vi "Select PPMS Class.vi"(8 "error in (no error)":errorcluster, 11 "Select PPMS":T1) -> (0 "error out":errorcluster, 3 "instrument.PPMS out":refnum<class "instrument.PPMS.lvclass">)   [LabVIEW 2019, in "instrument.PPMS.lvclass"]
uses:
  instrument.PPMS.lvclass
  Typedefs/Select PPMS--Enum.ctl
  instrument.PPMS1/instrument.PPMS1.lvclass
  C:/Users/patrick/Documents/GitHub/PPMS-Monitor-and-Control/lvsrc/instrument.PPMS/instrument.PPMS.lvclass
  instrument.PPMS2/instrument.PPMS2.lvclass
  instrument.PPMS3/instrument.PPMS3.lvclass
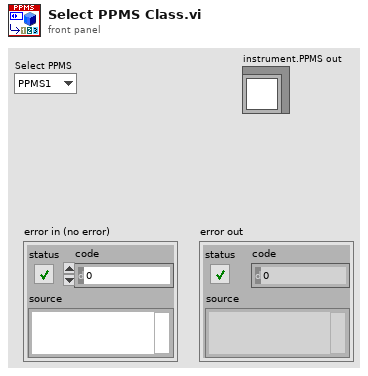
[diagram p1: front panel]
types:
  T1 = typedef "instrument.PPMS.lvclass/Select PPMS--Enum.ctl" = enum16{"PPMS1", "PPMS2", "PPMS3", "simulate"}
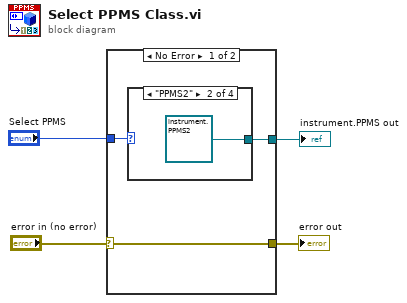
[diagram p0: block diagram]
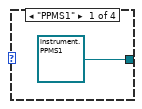
[diagram p2: hidden frame]
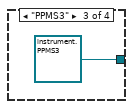
[diagram p3: hidden frame]
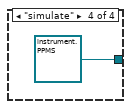
[diagram p4: hidden frame]
diagram:
  n1 = case shown="No Error" "error in (no error)" {
    selector: "error in (no error)" -> [w5 w12]
    tunnel: [w7 _] -> w4
    tunnel: "Select PPMS" -> [w6 _]
    tunnel: [w5 w12] -> w1
    frame No Error {
      n2 = case shown="\"PPMS2\"" w6 {
        tunnel: [refnum<class "instrument.PPMS1.lvclass"> refnum ("instrument.PPMS1.lvclass") refnum<class "instrument.PPMS2.lvclass"> refnum ("instrument.PPMS2.lvclass") refnum<class "instrument.PPMS3.lvclass"> refnum ("instrument.PPMS3.lvclass") refnum<class "instrument.PPMS.lvclass"> refnum ("instrument.PPMS2.lvclass")] -> w7
        frame "PPMS1" {
        }
        frame "PPMS2" {
        }
        frame "PPMS3" {
        }
        frame "simulate" {
        }
      }
    }
    frame Error {
    }
  }
  "instrument.PPMS out" <- w4
  "error out" <- w1
